vi "Voltages.vi"(11 "file path (dialog if empty)":path) -> ()   [LabVIEW 2014]
uses:
  <vilib>/Utility/file.llb/Write To Spreadsheet File (DBL).vi
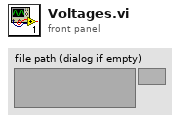
[diagram p1: front panel]
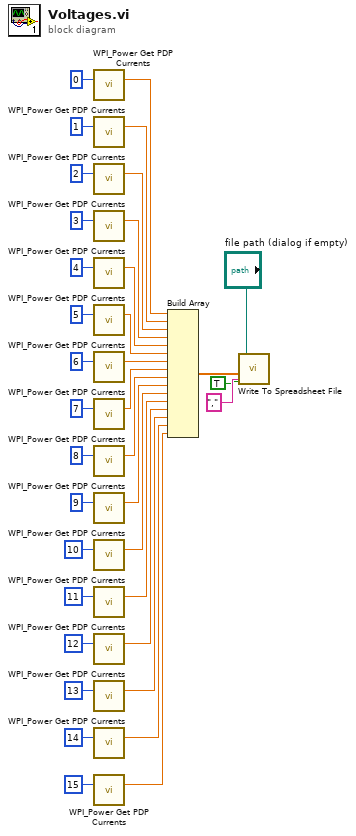
[diagram p0: block diagram]
diagram:
  n1 = call <vilib>:"WPI_Power Get PDP Currents.vi"("PDP Channel"=0) -> ("current (A)"=w32:dbl)  [unwired: 12 in, 2 out]
  n2 = call <vilib>:"WPI_Power Get PDP Currents.vi"("PDP Channel"=1) -> ("current (A)"=w30:dbl)  [unwired: 12 in, 2 out]
  n3 = call <vilib>:"WPI_Power Get PDP Currents.vi"("PDP Channel"=2) -> ("current (A)"=w28:dbl)  [unwired: 12 in, 2 out]
  n4 = call <vilib>:"WPI_Power Get PDP Currents.vi"("PDP Channel"=3) -> ("current (A)"=w26:dbl)  [unwired: 12 in, 2 out]
  n5 = call <vilib>:"WPI_Power Get PDP Currents.vi"("PDP Channel"=4) -> ("current (A)"=w24:dbl)  [unwired: 12 in, 2 out]
  n6 = call <vilib>:"WPI_Power Get PDP Currents.vi"("PDP Channel"=5) -> ("current (A)"=w22:dbl)  [unwired: 12 in, 2 out]
  n7 = call <vilib>:"WPI_Power Get PDP Currents.vi"("PDP Channel"=6) -> ("current (A)"=w20:dbl)  [unwired: 12 in, 2 out]
  n8 = call <vilib>:"WPI_Power Get PDP Currents.vi"("PDP Channel"=7) -> ("current (A)"=w18:dbl)  [unwired: 12 in, 2 out]
  n9 = call <vilib>:"WPI_Power Get PDP Currents.vi"("PDP Channel"=8) -> ("current (A)"=w16:dbl)  [unwired: 12 in, 2 out]
  n10 = call <vilib>:"WPI_Power Get PDP Currents.vi"("PDP Channel"=9) -> ("current (A)"=w14:dbl)  [unwired: 12 in, 2 out]
  n11 = call <vilib>:"WPI_Power Get PDP Currents.vi"("PDP Channel"=10) -> ("current (A)"=w12:dbl)  [unwired: 12 in, 2 out]
  n12 = call <vilib>:"WPI_Power Get PDP Currents.vi"("PDP Channel"=11) -> ("current (A)"=w10:dbl)  [unwired: 12 in, 2 out]
  n13 = call <vilib>:"WPI_Power Get PDP Currents.vi"("PDP Channel"=12) -> ("current (A)"=w8:dbl)  [unwired: 12 in, 2 out]
  n14 = call <vilib>:"WPI_Power Get PDP Currents.vi"("PDP Channel"=13) -> ("current (A)"=w5:dbl)  [unwired: 12 in, 2 out]
  n15 = call <vilib>:"WPI_Power Get PDP Currents.vi"("PDP Channel"=14) -> ("current (A)"=w4:dbl)  [unwired: 12 in, 2 out]
  n16 = call <vilib>:"WPI_Power Get PDP Currents.vi"("PDP Channel"=15) -> ("current (A)"=w2:dbl)  [unwired: 12 in, 2 out]
  n17 = Build Array(w32, w30, w28, w26, w24, w22, w20, w18, w16, w14, w12, w10, w8, w5, w4, w2) -> (w33:dbl[])
  n18 = call-poly <vilib>:"Write To Spreadsheet File.vi"("delimiter (\\t)"="," ("delimiter (\\t)"), "append to file? (new file:F)"=TRUE, "1D data"=w33, "file path (dialog if empty)"="file path (dialog if empty)") -> ()  [unwired: 4 in, 1 out]
